vi "ROM Test.vi"(11 "ROMFail":bool) -> (0 "error out":errorcluster, 3 "Result":bool)   [LabVIEW 2011]
doc: "Tests the Read Only Memory (ROM) on the motherboard."
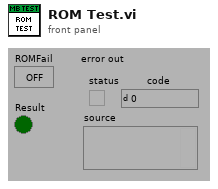
[diagram p1: front panel]
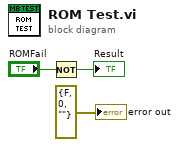
[diagram p0: block diagram]
diagram:
  n1 = Not(x="ROMFail") -> (.not. x?=→"Result":bool)
  "error out" <- errorcluster {"status"=FALSE, "code"=0, "source"=""} ("error out")
